vi "FLOM Test Program.vi"() -> ()   [LabVIEW 2018, in "FLOM Pump.lvlib"]
uses:
  FLOM Pump.lvlib
  Settings Cluster.ctl
panel:
  in  "stop":bool
  out "Pressure":dbl
  out "Flow Rate":dbl
  out "Connection Error":bool
  out "No Pump Connected":bool
  out "Pump On?":enum16{"Off", "On", "Not Initialized"}(ring)
  in  "Speed":dbl
  in  "VICI Settings":T1={"VISA resource name"="COM4", "Simulated?"=FALSE, "Pump Number"=1.0}
  in  "Pause":bool
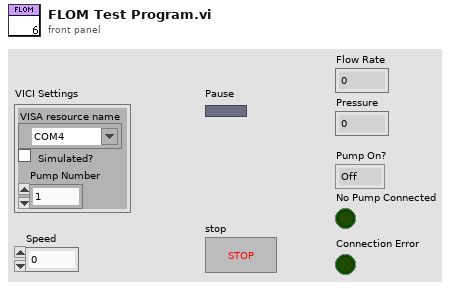
[diagram p1: front panel]
types:
  T1 = typedef "FLOM Pump.lvlib/Settings Cluster.ctl" = cluster{"VISA resource name":refnum<visa-resource-name>, "Simulated?":bool, "Pump Number":dbl}
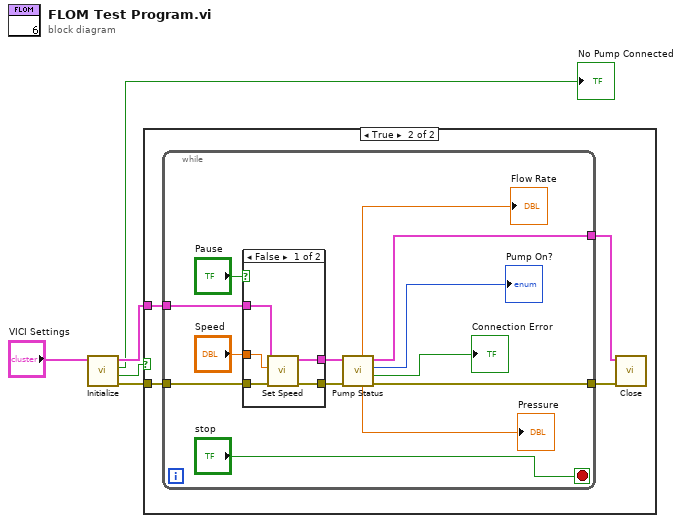
[diagram p0: block diagram]
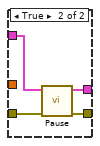
[diagram p3: hidden frame]
diagram:
  n1 = call "Initialize.vi"("FLOM Settings in"="VICI Settings") -> ("error out"=w3:errorcluster, "Initialized"=w2:bool, "No Pump Connected"=→"No Pump Connected":bool, "FLOM Settings out"=w4:T1)  [unwired: 7 in]
  n2 = case shown="True" w2 {
    tunnel: w4 -> [_ w9]
    tunnel: w3 -> [_ w8]
    frame False {
    }
    frame True {
      n3 = while {
        tunnel: w9 -> [w21]
        tunnel: w8 -> [w20]
        tunnel: [w17] -> w7
        tunnel: [w16] -> w6
        stop <- "stop" stop-if-true
        n4 = case shown="False" "Pause" {
          tunnel: w21 -> [w27 w29]
          tunnel: w20 -> [w26 w28]
          tunnel: [w25 w30] -> w19
          tunnel: [w24 w31] -> w18
          tunnel: "Speed" -> [w23 _]
          frame False {
            n5 = call "Set Speed.vi"("error in (no error)"=w26, "speed"=w23, "FLOM Settings in"=w27) -> ("error out"=w25:errorcluster, "FLOM Settings out"=w24:T1)  [unwired: 6 in, 1 out]
          }
          frame True {
            n6 = call "Pause.vi"("error in (no error)"=w28, "FLOM Settings in"=w29) -> ("error out"=w30:errorcluster, "FLOM Settings out"=w31:T1)  [unwired: 8 in]
          }
        }
        n7 = call "Pump Status.vi"("error in (no error)"=w19, "FLOM Settings In"=w18) -> ("error out"=w16:errorcluster, "Connection Error"=→"Connection Error":bool, "Pump On?"=→"Pump On?":enum16{"Off", "On", "Not Initialized"}, "FLOM Settings Out"=w17:T1, "Pressure"=→"Pressure":dbl, "Flow Rate"=→"Flow Rate":dbl)  [unwired: 4 in]
      }
      n8 = call "Close.vi"("error in (no error)"=w6, "FLOM Settings in"=w7) -> ()  [unwired: 8 in, 2 out]
    }
  }
